vi "Images processed counts.vi"(10 "Imaging data processed in":u32, 11 "output valid":bool) -> (3 "Imaging data processed out":u32)   [LabVIEW 2015]
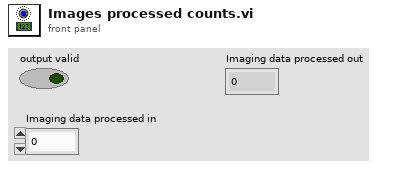
[diagram p1: front panel]
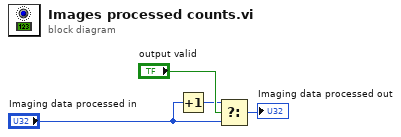
[diagram p0: block diagram]
diagram:
  n1 = Increment(x="Imaging data processed in") -> (x+1=w2:u32)
  n2 = Select(t=w2, s="output valid", f="Imaging data processed in") -> (s? t:f=→"Imaging data processed out":u32)
